vi "Data cloning (SubVI).vi"(8 "error in (no error)":errorcluster, 10 "File/folder path":path[](array[path]), 11 "USB drive's list":path[](array[path])) -> (0 "error out":errorcluster)   [LabVIEW 2018]
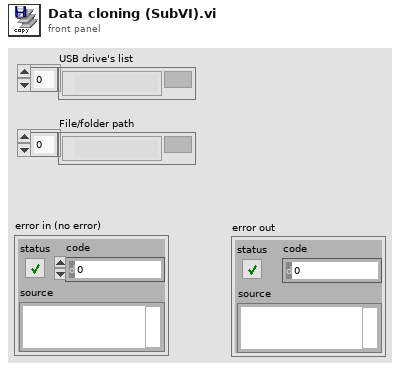
[diagram p1: front panel]
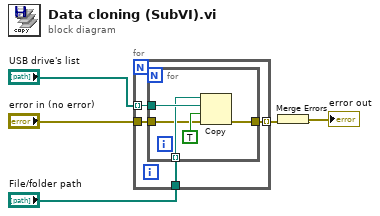
[diagram p0: block diagram]
diagram:
  n1 = for {
    tunnel: "USB drive's list" -> [w9] mode=indexing
    tunnel: [w8] -> w3 mode=indexing
    tunnel: "File/folder path" -> [w7]
    tunnel: "error in (no error)" -> [w6]
    n2 = for {
      tunnel: w9 -> [w14]
      tunnel: [w13] -> w8
      tunnel: w7 -> [w11] mode=indexing
      tunnel: w6 -> [w10]
      n3 = Copy(8:w10, 9:TRUE ("overwrite (F)"), 10:w14, 11:w11) -> (0:w13:errorcluster)  [unwired: 1 in, 2 out]
    }
  }
  n4 = Merge Errors(w3) -> (→"error out":errorcluster)
